vi "Configure Voltage Level.vi"(8 "error in (no error)":errorcluster, 9 "Level (0.0 Volts)":dbl format="%.2p", 11 "VISA resource name":refnum<visa-resource-name>) -> (0 "error out":errorcluster, 3 "VISA resource name out":refnum<visa-resource-name>)   [LabVIEW 2018, in "Agilent E364X Series.lvlib"]
doc: "This VI configures the DC voltage level the power supply attempts to generate."
uses:
  Agilent E364X Series.lvlib
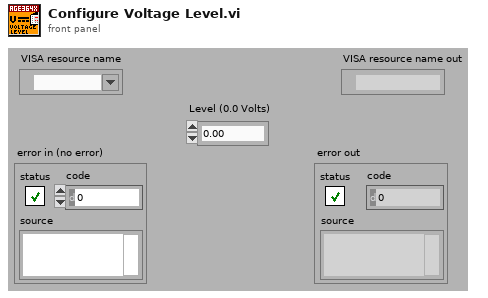
[diagram p1: front panel]
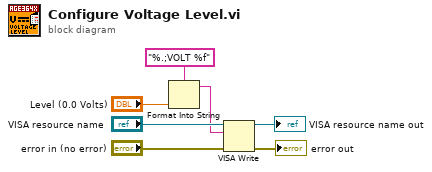
[diagram p0: block diagram]
diagram:
  n1 = Format Into String(format string="%.;VOLT %f", "Level (0.0 Volts)") -> (resulting string=w3:string)  [unwired: 2 in, 1 out]
  n2 = VISA Write(VISA resource name="VISA resource name", write buffer=w3, error in (no error)="error in (no error)") -> (VISA resource name out=→"VISA resource name out":refnum<visa-resource-name>, error out=→"error out":errorcluster)  [unwired: 1 out]
